vi "Latch.vi"(1 "Input":bool) -> (0 "Output":bool)   [LabVIEW 2014]
doc: "This VI holds a true value for 1 cycle after the true is released to false. In a real life button press this would hld true one cycle after the button is released and hold false in all other cases. Suggested implementation would be a bump for a motor."
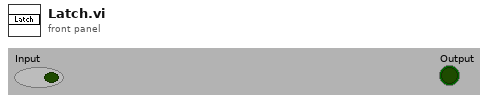
[diagram p1: front panel]
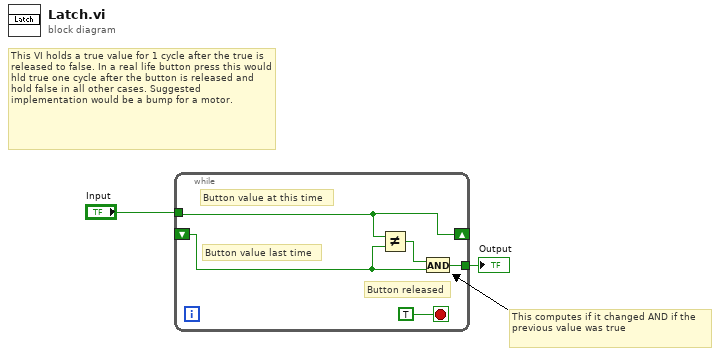
[diagram p0: block diagram]
diagram:
  # "This computes if it changed AND if the previous value was true"
  # "This VI holds a true value for 1 cycle after the true is released to false. In a real life button press this would hld true one cycle after the button is released and hold false in all other cases. Suggested implementation would be a bump for a motor."
  n1 = while {
    tunnel: [w6] -> w1
    tunnel: "Input" -> [w5]
    shift-right: [w5] -> _
    shift-left: _ -> [w4]
    stop <- TRUE ("stop") stop-if-true
    # "Button released"
    # "Button value last time"
    # "Button value at this time"
    n2 = Not Equal?(x=w5, y=w4) -> (x != y?=w7:bool)
    n3 = And(x=w7, y=w4) -> (x .and. y?=w6:bool)
  }
  "Output" <- w1
